vi "Release DOM Ref.vi"(8 "error in":errorcluster, 11 "System in":refnum<class "System.lvclass">) -> (0 "error out":errorcluster, 3 "System out":refnum<class "System.lvclass">)   [LabVIEW 2014, in "System.lvclass"]
uses:
  System.lvclass
  <vilib>/xml/Close Reference(Node).vi
  <vilib>/xml/NI_XML.lvlib
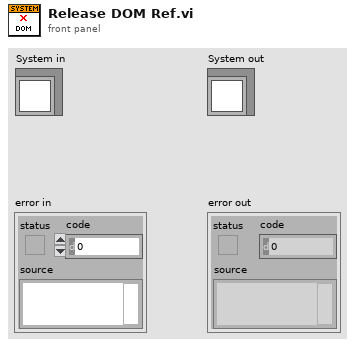
[diagram p1: front panel]
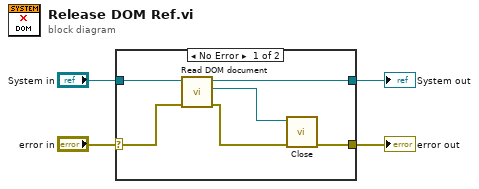
[diagram p0: block diagram]
diagram:
  n1 = case shown="No Error" "error in" {
    selector: "error in" -> [w6 w12]
    tunnel: [w7 w12] -> w3
    tunnel: [w9 w11] -> w1
    tunnel: "System in" -> [w10 w11]
    frame No Error {
      n2 = call-dynamic "Read DOM document.vi"("error in"=w6, "System in"=w10) -> ("error out"=w5:errorcluster, "DOM document"=w8:refnum<k20>, "System out"=w9:refnum<class "System.lvclass">)  [unwired: 7 in]
      n3 = call-poly <vilib>:"Close.vi"("error in (no error)"=w5, "node"=w8) -> ("error out"=w7:errorcluster)  [unwired: 7 in]
    }
    frame Error {
    }
  }
  "error out" <- w3
  "System out" <- w1
